vi "daq 1.vi"() -> ()   [LabVIEW 2025]
panel:
  in  "stop":bool
  in  "stop (T)":bool=TRUE
  out "Waveform Graph":dynamicdata(graph)
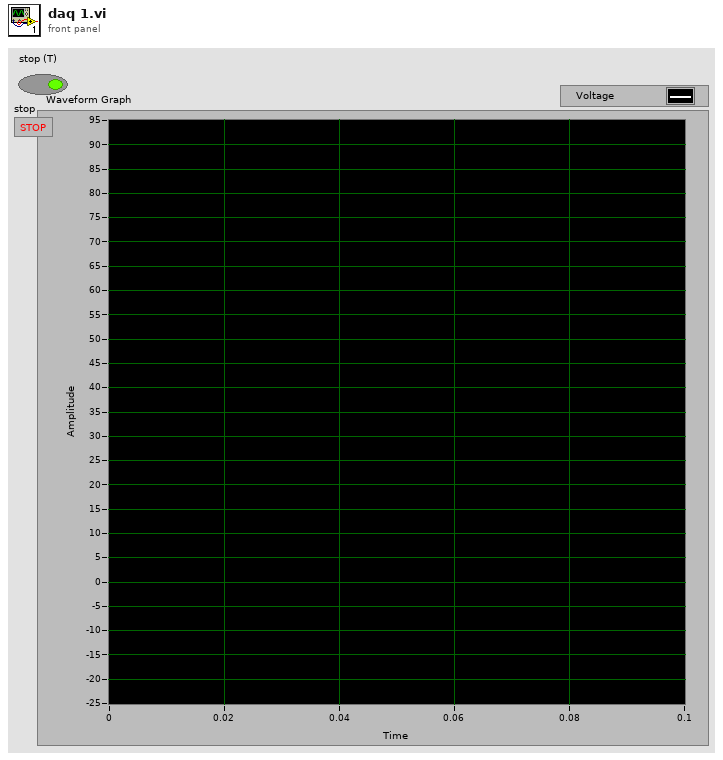
[diagram p1: front panel]
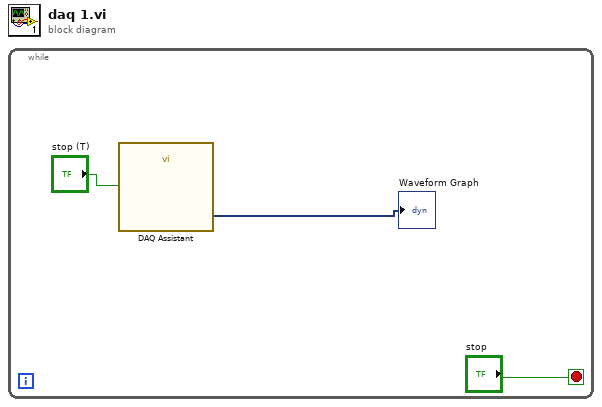
[diagram p0: block diagram]
diagram:
  n1 = while {
    stop <- "stop" stop-if-true
    n2 = call "DAQ Assistant"("stop (T)"="stop (T)") -> ("data"=→"Waveform Graph":dynamicdata)  [unwired: 16 in, 2 out]
  }
